vi "niScope Close Virtual Channels.vi"(8 "error in":errorcluster, 11 "niScope in":T1={"channel cfg"=[], "sessions"=[], "multi cards"=FALSE, "channels"=0, "type"=enum."n/a", "memory [B/chn]"=0, "ext. clock [Hz]"=0.0, "samples count"=0, "use streaming"=FALSE, "proc setup"={"packet size [smpl]"=0, "current timeout [s]"=0.0, "blk2blk timeout [s]"=0.0, "event time"=timestamp(0 s since 1904-01-01), "temp sampl T [s]"=0.0, "data queue"=refnum, "stop notifier"=refnum, "proc ref"=refnum}, "sample width [B]"=0, "ranges [V]"=[], "trigger setup"={"coupling"=1, "level [V]"=0.0, "slope"=0, "mode"=enum."Immediate"}, "fs [Hz]"=0.0} {"trigger setup"."level [V]" format="%.2f"; "trigger setup"."coupling" items=["AC"=0, "DC"=1, "HF Reject"=3, "LF Reject"=4, "AC Plus HF Reject"=1001]; "channel cfg"."Range [Vpk]" min=0.0; "channel cfg"."Channel" min=0}) -> (0 "error out":errorcluster, 3 "niScope out":T1={"channel cfg"=[], "sessions"=[], "multi cards"=FALSE, "channels"=0, "type"=enum."n/a", "memory [B/chn]"=0, "ext. clock [Hz]"=0.0, "samples count"=0, "use streaming"=FALSE, "proc setup"={"packet size [smpl]"=0, "current timeout [s]"=0.0, "blk2blk timeout [s]"=0.0, "event time"=timestamp(0 s since 1904-01-01), "temp sampl T [s]"=0.0, "data queue"=refnum, "stop notifier"=refnum, "proc ref"=refnum}, "sample width [B]"=0, "ranges [V]"=[], "trigger setup"={"coupling"=1, "level [V]"=0.0, "slope"=0, "mode"=enum."Immediate"}, "fs [Hz]"=0.0} {"trigger setup"."level [V]" format="%.2f"; "trigger setup"."coupling" items=["AC"=0, "DC"=1, "HF Reject"=3, "LF Reject"=4, "AC Plus HF Reject"=1001]; "channel cfg"."Range [Vpk]" min=0.0; "channel cfg"."Channel" min=0})   [LabVIEW 2013, in "niScope Virtual Digitizer.lvlib"]
doc: "Close all virtual channels. Executes even if error is on the input. Call this after the measurement is done and ADC not needed anymore."
uses:
  niScope Virtual Digitizer.lvlib
  niScope Session.ctl
  niScope Virtual Channel Config.ctl
  niScope Virtual Channel Mode.ctl
  niScope Virtual Channel Input Z.ctl
  niScope Virtual Channel Coupling.ctl
  niScope Type.ctl
  niScope Digitizing Process Options.ctl
  niScope Data Packet.ctl
  niScope Trigger Setup.ctl
  <instrlib>/niScope/Controls/niScope trigger coupling.ctl
  <instrlib>/niScope/Controls/niScope trigger slope.ctl
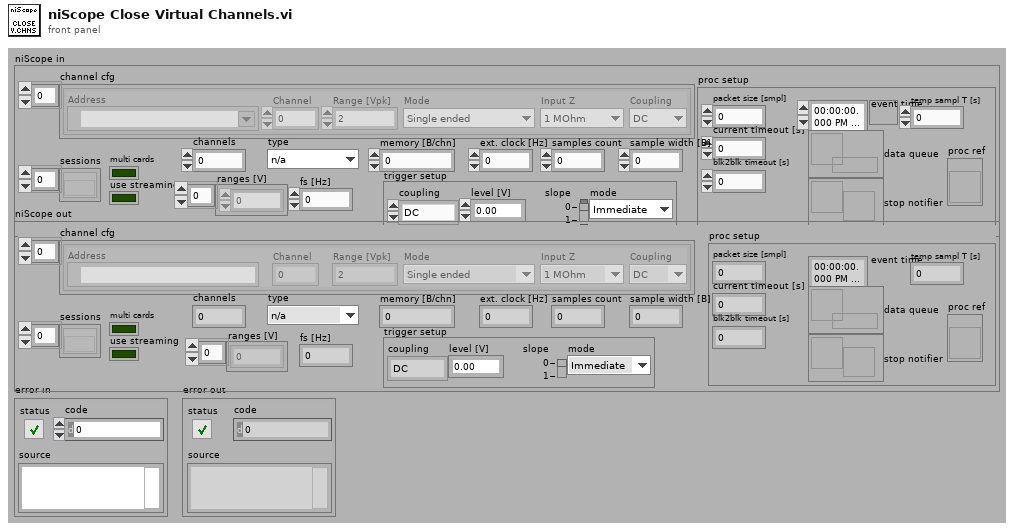
[diagram p1: front panel]
types:
  T1 = typedef "niScope Virtual Digitizer.lvlib/niScope Session.ctl" = cluster{"channel cfg":T2[], "sessions":refnum<k20>[], "multi cards":bool, "channels":i32, "type":T6, "memory [B/chn]":i32, "ext. clock [Hz]":dbl, "samples count":i64, "use streaming":bool, "proc setup":T7, "sample width [B]":i32, "ranges [V]":dbl[], "trigger setup":T8, "fs [Hz]":dbl}
  T2 = typedef "niScope Virtual Digitizer.lvlib/niScope Virtual Channel Config.ctl" = cluster{"Address":refnum<k15>, "Channel":i32, "Mode":T3, "Input Z":T4, "Coupling":T5, "Range [Vpk]":dbl}
  T3 = typedef "niScope Virtual Digitizer.lvlib/niScope Virtual Channel Mode.ctl" = enum16{"Single ended", "Unbal. differential", "Differential"}
  T4 = typedef "niScope Virtual Digitizer.lvlib/niScope Virtual Channel Input Z.ctl" = enum16{"1 MOhm", "50 Ohm"}
  T5 = typedef "niScope Virtual Digitizer.lvlib/niScope Virtual Channel Coupling.ctl" = enum16{"AC", "DC", "GND"}
  T6 = typedef "niScope Virtual Digitizer.lvlib/niScope Type.ctl" = enum16{"n/a", "5922"}
  T7 = typedef "niScope Virtual Digitizer.lvlib/niScope Digitizing Process Options.ctl" = cluster{"packet size [smpl]":i64, "current timeout [s]":dbl, "blk2blk timeout [s]":dbl, "event time":timestamp, "temp sampl T [s]":dbl, "data queue":refnum<queue>, "stop notifier":refnum<notifier>, "proc ref":refnum<vi>}
  T8 = typedef "niScope Virtual Digitizer.lvlib/niScope Trigger Setup.ctl" = cluster{"coupling":T9, "level [V]":dbl, "slope":T10, "mode":enum16{"Immediate", "External", "Level"}}
  T9 = typedef "niScope trigger coupling.ctl" = u16
  T10 = typedef "niScope trigger slope.ctl" = i32
  T11 = typedef "niScope Virtual Digitizer.lvlib/niScope Physical Cards.ctl" = cluster{"chn lst":i32[], "addr":refnum<k15>, "chn pos":i32[]}
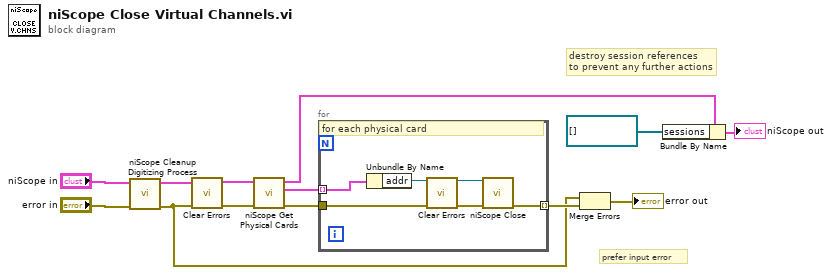
[diagram p0: block diagram]
diagram:
  # "destroy session references\nto prevent any further actions"
  # "prefer input error"
  n1 = call "niScope Cleanup Digitizing Process.vi"("error in"="error in", "niScope in"="niScope in") -> ("error out"=w1:errorcluster, "niScope out"=w3:T1)  [unwired: 8 in]
  n2 = call <vilib>:"Clear Errors.vi"("error in (no error)"=w1) -> ("error out"=w4:errorcluster)  [unwired: 6 in]
  n3 = call "niScope Get Physical Cards.vi"("error in"=w4, "niScope in"=w3) -> ("error out"=w12:errorcluster, "card list"=w11:T11[], "niScope out"=w8:T1)  [unwired: 7 in]
  n4 = for {
    tunnel: w11 -> [w17] mode=indexing
    tunnel: w12 -> [w16]
    tunnel: [w13] -> w10 mode=indexing
    # "for each physical card"
    n5 = Unbundle By Name(w17) -> ("addr"=w14:refnum<k15>)
    n6 = call <vilib>:"Clear Errors.vi"("error in (no error)"=w16) -> ("error out"=w15:errorcluster)  [unwired: 6 in]
    n7 = call <instrlib>:"niScope Close.vi"("instrument handle"=w14, "error in"=w15) -> ("error out"=w13:errorcluster)  [unwired: 13 in]
  }
  n8 = Merge Errors(w1, w10) -> (→"error out":errorcluster)
  n9 = Bundle By Name(cluster=w8, "sessions"=refnum<k20>[] []) -> (→"niScope out":T1)
